vi "Assert Class Serialize.vi"() -> ()   [LabVIEW 2015, in "Admin_Actor.lvlib" / "AttendRecord.lvclass"]
uses:
  AttendRecord.lvclass
  AttendRecord.lvclass/AttendRecord.ctl
panel:
  out "Name(\"\")":string
  out "data":refnum<class "AttendRecord.lvclass">
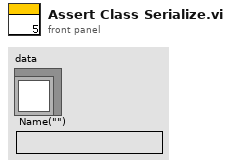
[diagram p1: front panel]
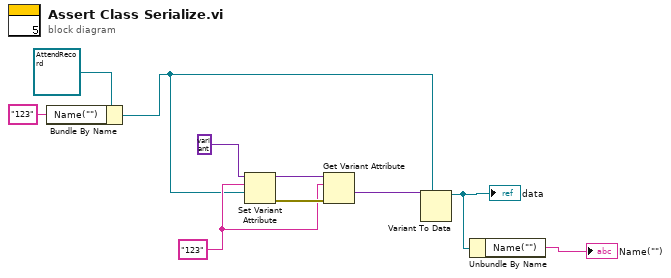
[diagram p0: block diagram]
diagram:
  w7 = "123" ("name")
  n1 = Bundle By Name(cluster=refnum<class "AttendRecord.lvclass"> refnum ("Admin_Actor.lvlib:AttendRecord.lvclass"), "Name(\"\")"="123" ("Name(\"\")")) -> (w4:refnum<class "AttendRecord.lvclass">)
  n2 = Set Variant Attribute(Variant=variant, name=w7, value=w4) -> (Variant out=w9:variant, error out=w8:errorcluster)  [unwired: 1 in, 1 out]
  n3 = Get Variant Attribute(Variant=w9, name=w7, error in=w8) -> (value=w6:variant)  [unwired: 1 in, 3 out]
  n4 = Variant To Data(type=w4, Variant=w6) -> (data=w2:refnum<class "AttendRecord.lvclass">)  [unwired: 1 in, 1 out]
  "data" <- w2
  n5 = Unbundle By Name(w2) -> ("Name(\"\")"=→"Name(\"\")":string)
